vi "extract to time range.vi"(6 "most recent?":bool, 7 "recent interval":dbl=5.0, 9 "t0":dbl=-1.0, 10 "t1":dbl=-1.0, 11 "elements":T1[](array[typedef])) -> (2 "extracted data":T1[](array[typedef]))   [LabVIEW 2017]
uses:
  typedefs/reading.ctl
  typedefs/readingType.ctl
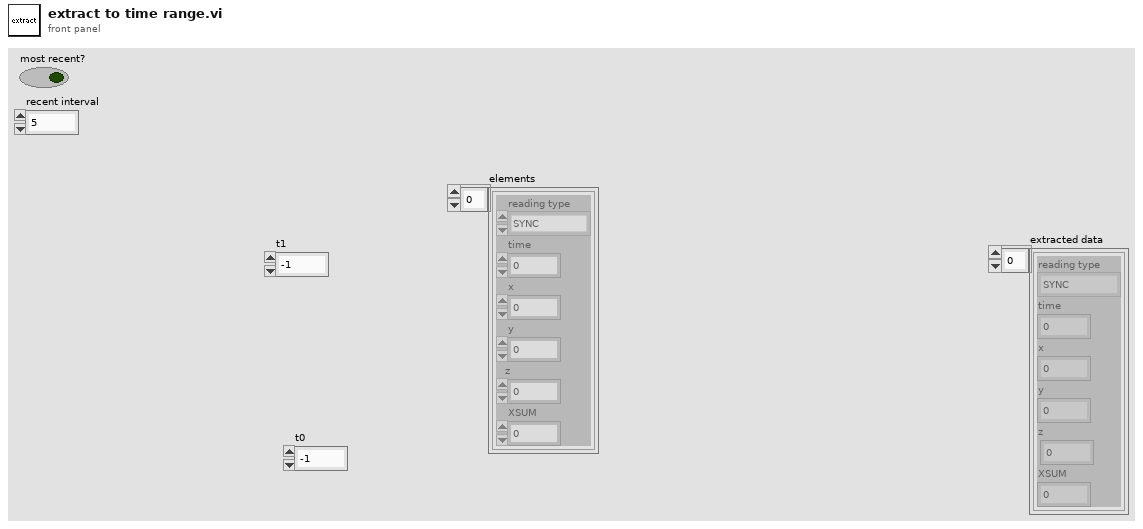
[diagram p1: front panel]
types:
  T1 = typedef "reading.ctl" = cluster{"reading type":T2, "time":fxp<+,48,48>, "x":sgl, "y":sgl, "z":sgl, "XSUM":u8}
  T2 = typedef "readingType.ctl" = enum8{"SYNC", "DETVAL", "COILI", "MAGVEC", "ACCVEC", "CROSSING", "MAGVEC0", "MAGVEC1", "MAGVEC2", "MAGVEC3", "MAGVEC4", "MAGVEC5", "MAGVEC6", "MAGVEC7"}
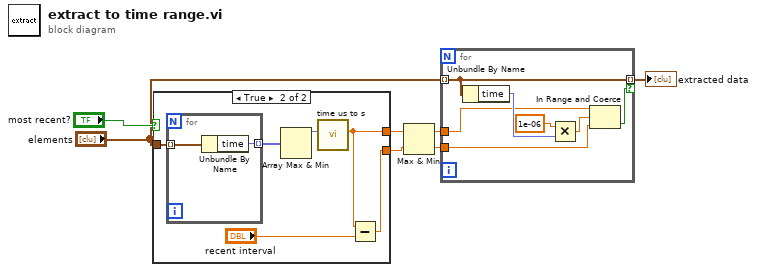
[diagram p0: block diagram]
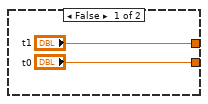
[diagram p2: hidden frame]
diagram:
  n1 = case shown="True" "most recent?" {
    tunnel: "elements" -> [_ w15]
    tunnel: ["t1" w11] -> w2
    tunnel: ["t0" w10] -> w1
    frame False {
    }
    frame True {
      n2 = for {
        tunnel: w15 -> [w17] mode=indexing
        tunnel: [w16] -> w14 mode=indexing
        n3 = Unbundle By Name(w17) -> ("time"=w16:fxp<+,48,48>)
      }
      n4 = Array Max & Min(array=w14) -> (max value=w13:fxp<+,48,48>)  [unwired: 3 out]
      n5 = call "time us to s.vi"("time (us)"=w13) -> ("time (s)"=w11:dbl)  [unwired: 10 in]
      n6 = Subtract(x=w11, y="recent interval") -> (x-y=w10:dbl)
    }
  }
  n7 = Max & Min(x=w2, y=w1) -> (max(x,y)=w6:dbl, min(x,y)=w5:dbl)
  n8 = for {
    tunnel: "elements" -> [w24] mode=indexing
    tunnel: [w24] -> w7 mode=indexing if=w20
    tunnel: w6 -> [w22]
    tunnel: w5 -> [w21]
    n9 = Unbundle By Name(w24) -> ("time"=w23:fxp<+,48,48>)
    n10 = Multiply(x=1e-06, y=w23) -> (x*y=w19:dbl)
    n11 = In Range and Coerce(upper limit=w22, x=w19, lower limit=w21) -> (In Range?=w20:bool)  [unwired: 1 out]
  }
  "extracted data" <- w7
